vi "format-input.vi"(10 "tasks":T2[](array[typedef])) -> (1 "HTML":string[](array[string]), 2 "states":T1[](array[typedef]))   [LabVIEW 2014]
uses:
  controls/state program.ctl
  controls/state-machine.ctl
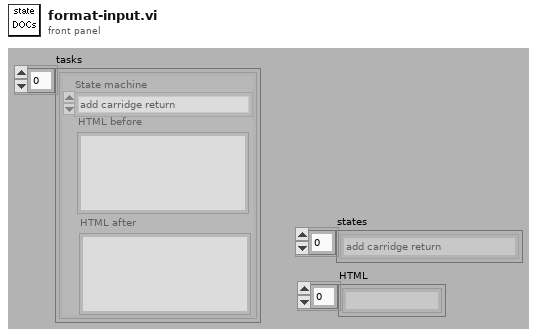
[diagram p1: front panel]
types:
  T1 = typedef "state-machine.ctl" = enum16{"add carridge return", "init", "Read-inputs", "edit generated file", "end", "Add front panel", "Add Block Diagram", "Add VI icon", "Add VI description", "Add VI hiearchy", "Add list of sub vis", "add custom html", "open report in browser", "Save report to file", "dispose report", "Add header text", "Create style .css", "add-red-box-header", "Delete Temp Files", "Remove-path-element", "add-revision-history", "add-icon-image-only"}
  T2 = typedef "state program.ctl" = cluster{"State machine":T1, "HTML before":string, "HTML after":string}
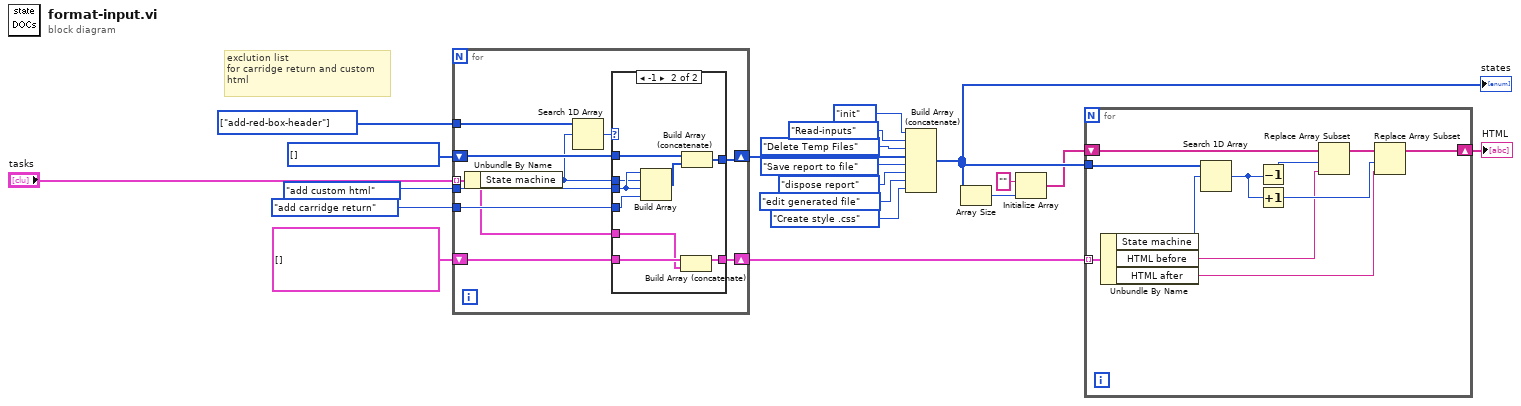
[diagram p0: block diagram]
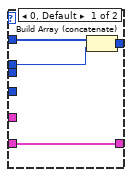
[diagram p2: hidden frame]
diagram:
  w20 = T1[] [enum."add-red-box-header"] items=["add carridge return", "init", "Read-inputs", "edit generated file", "end", "Add front panel", "Add Block Diagram", "Add VI icon", "Add VI description", "Add VI hiearchy", "Add list of sub vis", "add custom html", "open report in browser", "Save report to file", "dispose report", "Add header text", "Create style .css", "add-red-box-header", "Delete Temp Files", "Remove-path-element", "add-revision-history", "add-icon-image-only"]
  w5 = T1[] [] items=["add carridge return", "init", "Read-inputs", "edit generated file", "end", "Add front panel", "Add Block Diagram", "Add VI icon", "Add VI description", "Add VI hiearchy", "Add list of sub vis", "add custom html", "open report in browser", "Save report to file", "dispose report", "Add header text", "Create style .css", "add-red-box-header", "Delete Temp Files", "Remove-path-element", "add-revision-history", "add-icon-image-only"]
  # "exclution list\nfor carridge return and custom\nhtml"
  n1 = for {
    tunnel: "tasks" -> [w21] mode=indexing
    tunnel: state-machine."add custom html" ("State machine") -> [w27]
    tunnel: state-machine."add carridge return" ("State machine") -> [w30]
    shift-right: [w28] -> w15
    shift-left: w5 -> [w29]
    tunnel: w20 -> [w24]
    shift-right: [w23] -> w4
    shift-left: T2[] [] -> [w22]
    n2 = Unbundle By Name(w21) -> ("State machine"=w26:T1)
    n3 = Search 1D Array(1D array=w24, element=w26) -> (index of element=w25:i32)  [unwired: 1 out]
    n4 = case shown="-1" w25 {
      tunnel: w30 -> [_ w43]
      tunnel: w29 -> [w34 w41]
      tunnel: [w33 w40] -> w28
      tunnel: w26 -> [w32 w38]
      tunnel: w27 -> [_ w39]
      tunnel: [w31 w37] -> w23
      tunnel: w22 -> [w31 w36]
      tunnel: w21 -> [_ w35]
      frame 0, Default {
        n5 = Build Array (concatenate)(w34, w32) -> (w33:T1[])
      }
      frame -1 {
        n6 = Build Array(w39, w38, w39, w43) -> (w42:T1[])
        n7 = Build Array (concatenate)(w36, w35) -> (w37:T2[])
        n8 = Build Array (concatenate)(w41, w42) -> (w40:T1[])
      }
    }
  }
  n9 = Build Array (concatenate)(state-machine."init" ("element"), state-machine."Read-inputs" ("element"), state-machine."Delete Temp Files" ("element"), w15, state-machine."Save report to file" ("element"), state-machine."dispose report" ("element"), state-machine."edit generated file" ("element"), state-machine."Create style .css" ("element")) -> (w9:T1[])
  "states" <- w9
  n10 = Array Size(array=w9) -> (size(s)=w8:i32)
  n11 = Initialize Array("", w8) -> (w6:string[])
  n12 = for {
    tunnel: w9 -> [w54]
    tunnel: w4 -> [w53] mode=indexing
    shift-right: [w44] -> w2
    shift-left: w6 -> [w50]
    n13 = Unbundle By Name(w53) -> ("State machine"=w52:T1, "HTML before"=w46:string, "HTML after"=w45:string)
    n14 = Search 1D Array(1D array=w54, element=w52) -> (index of element=w51:i32)  [unwired: 1 out]
    n15 = Decrement(x=w51) -> (x-1=w48:i32)
    n16 = Increment(x=w51) -> (x+1=w47:i32)
    n17 = Replace Array Subset(array=w50, new element=w46, index=w48) -> (w49:string[])
    n18 = Replace Array Subset(array=w49, new element=w45, index=w47) -> (w44:string[])
  }
  "HTML" <- w2
